vi "Set High Pass Filter.vi"(9 "High Pass":u16(ring) items=["Off", "13 Hz", "104 Hz"], 11 "RS232":refnum<visa-resource-name>="ASRL27::INSTR") -> (0 "Success?":bool, 3 "RS232 out":refnum<visa-resource-name>="ASRL27::INSTR")   [LabVIEW 2022 SP3]
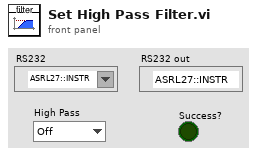
[diagram p1: front panel]
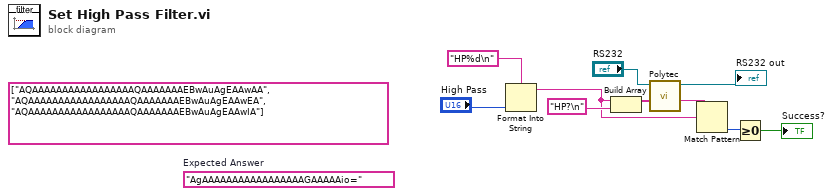
[diagram p0: block diagram]
diagram:
  (unwired) string[] ["AQAAAAAAAAAAAAAAAAAQAAAAAAAEBwAuAgEAAwAA", "AQAAAAAAAAAAAAAAAAAQAAAAAAAEBwAuAgEAAwEA", "AQAAAAAAAAAAAAAAAAAQAAAAAAAEBwAuAgEAAwIA"]
  (unwired) "AgAAAAAAAAAAAAAAAAAGAAAAAio="  # Expected Answer
  n1 = Format Into String(format string="HP%d\n", "High Pass") -> (resulting string=w1:string)  [unwired: 2 in, 1 out]
  n2 = Build Array(w1, "HP?\n" ("format string")) -> (w2:string[])
  n3 = call "Polytec.vi"("RS232"="RS232", "Strings"=w2) -> ("RS232 out"=→"RS232 out":refnum<visa-resource-name>, "String Read"=w5:string)  [unwired: 7 in]
  n4 = Match Pattern(string=w5, regular expression=w1) -> (offset past match=w6:i32)  [unwired: 1 in, 3 out]
  n5 = Greater Or Equal To 0?(x=w6) -> (x >= 0?=→"Success?":bool)
